vi "ke37xx Scan Trigger Control.vi"(0 "VISA Resource Name":refnum<visa-resource-name>, 5 "Action (0: Clearl)":enum16{"Clear", "Set"}(ring), 7 "Trigger Type (0: All)":enum16{"All", "Channel", "Measure", "Sequence"}(ring), 11 "error in (no error)":errorcluster) -> (4 "VISA Resource Name Out":refnum<visa-resource-name>, 15 "error out":errorcluster)   [LabVIEW 2009, in "Keithley 3700 Series.lvlib"]
doc: "This VI allows you to set or clear the scan trigger arm event detector."
uses:
  <instrlib>/Keithley 3706/Keithley 3700 Series.lvlib
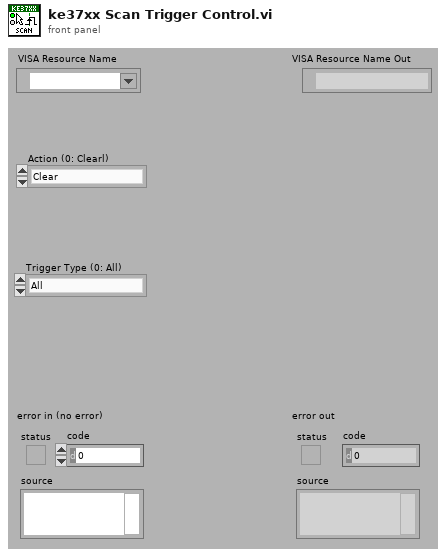
[diagram p1: front panel]
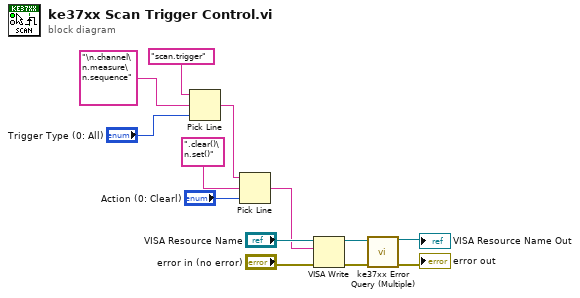
[diagram p0: block diagram]
diagram:
  n1 = Pick Line(string ("")="scan.trigger", multi-line string="\n.channel\n.measure\n.sequence", line index="Trigger Type (0: All)") -> (output string=w3:string)
  n2 = Pick Line(string ("")=w3, multi-line string=".clear()\n.set()", line index="Action (0: Clearl)") -> (output string=w5:string)
  n3 = VISA Write(VISA resource name="VISA Resource Name", write buffer=w5, error in (no error)="error in (no error)") -> (VISA resource name out=w9:refnum<visa-resource-name>, error out=w8:errorcluster)  [unwired: 1 out]
  n4 = call <instrlib>:"ke37xx Error Query (Multiple).vi"("VISA resource name"=w9, "error in (no error)"=w8) -> ("VISA resource name out"=→"VISA Resource Name Out":refnum<visa-resource-name>, "error out"=→"error out":errorcluster)  [unwired: 12 out]
